vi "Read Status.vi"(8 "error in (no error)":errorcluster, 10 "Status Register":T1(ring), 11 "VISA resource name":refnum<visa-resource-name>) -> (0 "error out":errorcluster, 2 "Register Bit":i16, 3 "VISA resource name out":refnum<visa-resource-name>)   [LabVIEW 2012, in "Temptronic TP04300.lvlib"]
doc: "This VI reads the Status Byte, Standard Event Status Register, Temperature Event Status Register, Temperature Event Condition Register and Auxiliary Condition Register.\n\nNote: Refer TP04300 instrument manual for bit assignment details."
uses:
  <instrlib>/Temptronic TP04300/Temptronic TP04300.lvlib
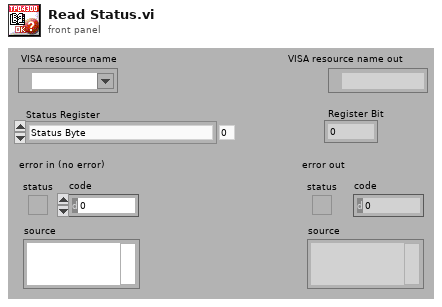
[diagram p1: front panel]
types:
  T1 = enum16{"Status Byte", "Standard Event Status Register", "Temperature Event Status Register", "Temperature Event Condition Register", "Auxiliary Condition Register"}
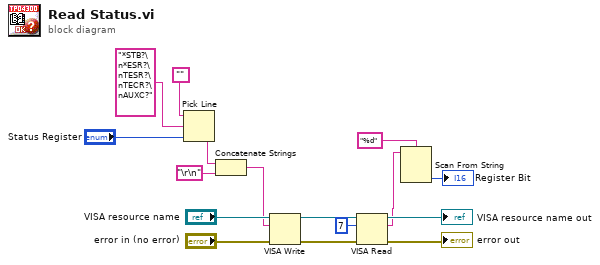
[diagram p0: block diagram]
diagram:
  n1 = Pick Line(string ("")="", multi-line string="*STB?\n*ESR?\nTESR?\nTECR?\nAUXC?", line index="Status Register") -> (output string=w3:string)
  n2 = Concatenate Strings(w3, "\r\n") -> (w4:string)
  n3 = VISA Write(VISA resource name="VISA resource name", write buffer=w4, error in (no error)="error in (no error)") -> (VISA resource name out=w14:refnum<visa-resource-name>, error out=w12:errorcluster)  [unwired: 1 out]
  n4 = VISA Read(VISA resource name=w14, byte count=u32 7, error in (no error)=w12) -> (VISA resource name out=→"VISA resource name out":refnum<visa-resource-name>, read buffer=w8:string, error out=→"error out":errorcluster)  [unwired: 1 out]
  n5 = Scan From String(format string="%d", input string=w8) -> (output 1=→"Register Bit":i16)  [unwired: 3 in, 3 out]
